vi "CRYImp wiz p1 file dialog.vi"(8 "error in (no error)":errorcluster, 10 "Main info cluster":T1, 11 "Page flags":T2) -> (0 "error out":errorcluster, 2 "Main info cluster out":T1, 3 "Page flags out":T2)   [LabVIEW 2013]
uses:
  Control/CRYImp wiz page flags.ctl
  Control/CRYImp wiz main info.ctl
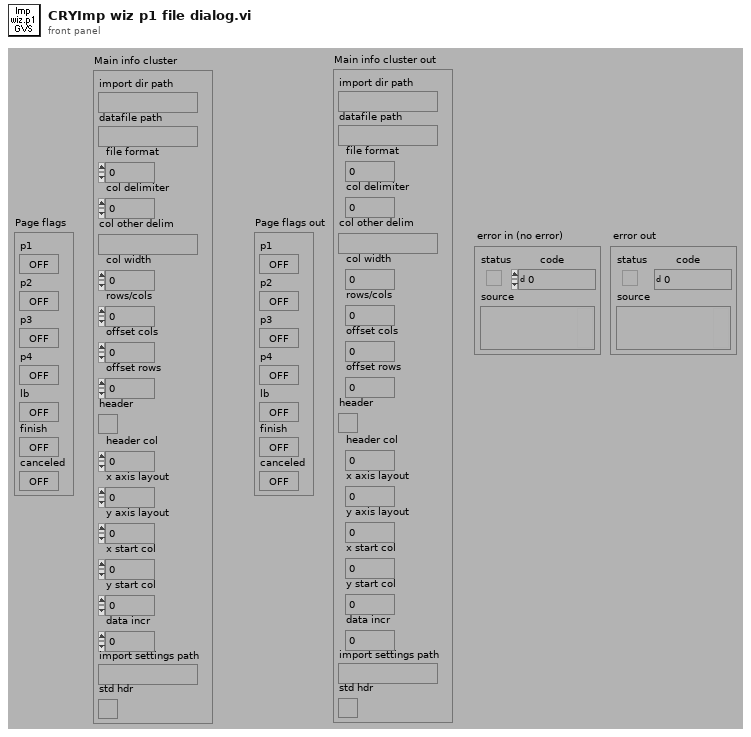
[diagram p1: front panel]
types:
  T1 = typedef "CRYImp wiz main info.ctl" = cluster{"import dir path":path, "datafile path":path, "file format":i32, "col delimiter":i32, "col other delim":string, "col width":i32, "rows/cols":i32, "offset cols":i32, "offset rows":i32, "header":bool, "header col":i32, "x axis layout":i32, "y axis layout":i32, "x start col":i32, "y start col":i32, "data incr":i32, "import settings path":path, "std hdr":bool}
  T2 = typedef "CRYImp wiz page flags.ctl" = cluster{"p1":bool, "p2":bool, "p3":bool, "p4":bool, "lb":bool, "finish":bool, "canceled":bool}
  T3 = enum32{"existing file", "new file", "new or existing file", "existing dir", "new dir", "new or existing dir", "existing file (use LLBs)", "new file (use LLBs)", "new or existing file (use LLBs)", "new or existing file or directory (use LLBs)", "existing dir (use LLBs)", "new dir (use LLBs)", "new or existing dir (use LLBs)", "existing file or dir", "new file or dir", "new or existing file or dir", "existing file or dir (use LLBs)", "new file or dir (use LLBs)"}
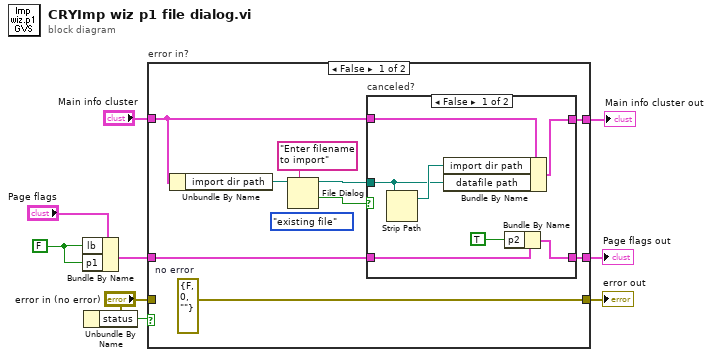
[diagram p0: block diagram]
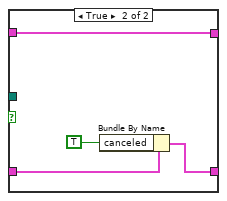
[diagram p2: hidden frame]
diagram:
  w3 = FALSE ("Bundle Element")
  n1 = Bundle By Name(cluster="Page flags", "lb"=w3, "p1"=w3) -> (w1:T2)
  n2 = Unbundle By Name("error in (no error)") -> ("status"=w5:bool)
  n3 = case "error in?" shown="False" w5 {
    tunnel: "Main info cluster" -> [w15 w30]
    tunnel: [w13 w30] -> w8
    tunnel: w1 -> [w12 w31]
    tunnel: [w11 w31] -> w7
    tunnel: "error in (no error)" -> [_ w32]
    tunnel: [w10 w32] -> w4
    frame False {
      w10 = errorcluster {"status"=FALSE, "code"=0, "source"=""}  # no error
      (unwired) T3."existing file" ("select mode (2)")
      n4 = Unbundle By Name(w15) -> ("import dir path"=w17:path)
      n5 = File Dialog(7:"Enter filename to import", 11:w17) -> (1:w16:bool, 3:w14:path)  [unwired: 1 in, 6 out]
      n6 = case "canceled?" shown="False" w16 {
        tunnel: w15 -> [w22 w29]
        tunnel: w14 -> [w24 _]
        tunnel: [w23 w29] -> w13
        tunnel: w12 -> [w21 w28]
        tunnel: [w19 w27] -> w11
        frame False {
          n7 = Strip Path(path=w24) -> (stripped path=w25:path)  [unwired: 1 out]
          n8 = Bundle By Name(cluster=w22, "import dir path"=w25, "datafile path"=w24) -> (w23:T1)
          n9 = Bundle By Name(cluster=w21, "p2"=TRUE ("Bundle Element")) -> (w19:T2)
        }
        frame True {
          n10 = Bundle By Name(cluster=w28, "canceled"=TRUE ("Bundle Element")) -> (w27:T2)
        }
      }
    }
    frame True {
    }
  }
  "Page flags out" <- w7
  "Main info cluster out" <- w8
  "error out" <- w4
